vi "FTW-ActorTemplate-RT-TopLevel.vi"() -> ()   [LabVIEW 2013]
uses:
  source/actor/Instance/FTW-ActorInstance.lvclass
  source/actor/Message/Base/FTW-Message.lvclass
  source/actor/Instance/FTW-ActorInstance.lvclass/FTW-ActorInstance.ctl
  source/actor/JobSequencer/FTW-SEQ-Current.vi
  source/actor/Message/Request/FTW-Message-IncomingRequest.lvclass
  source/actor/Ether/FTW-Ether.lvclass
panel:
  in  "Process Stop Button":bool
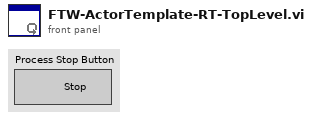
[diagram p1: front panel]
types:
  T1 = cluster{"Incoming Requests":refnum<event-registration>, "Local Messages":refnum<event-registration>, "Additional Registration Types":refnum<event-registration>}
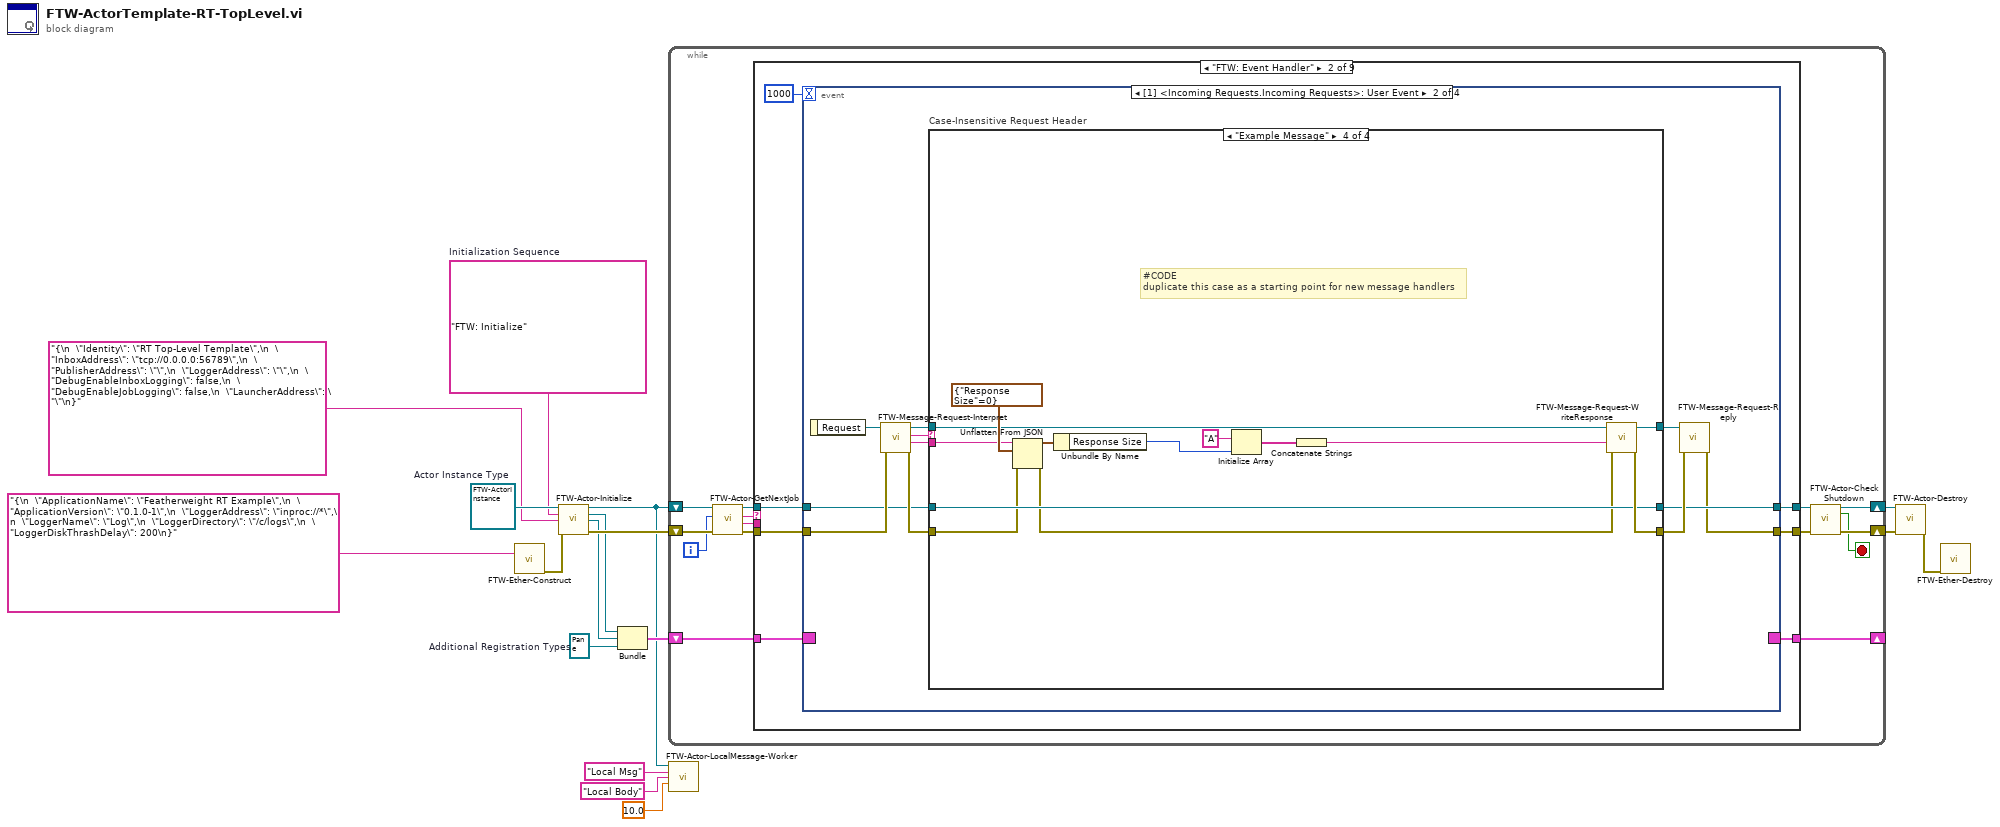
[diagram p0: block diagram]
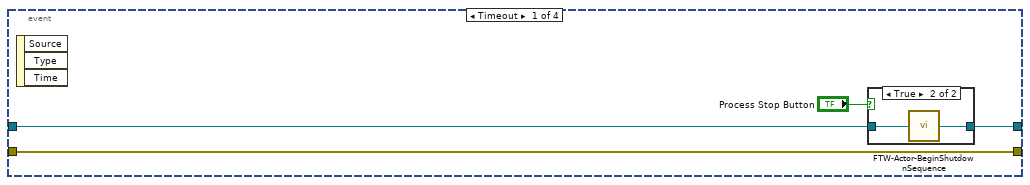
[diagram p3: hidden frame]
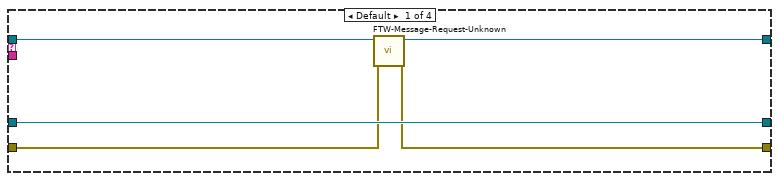
[diagram p5: hidden frame]
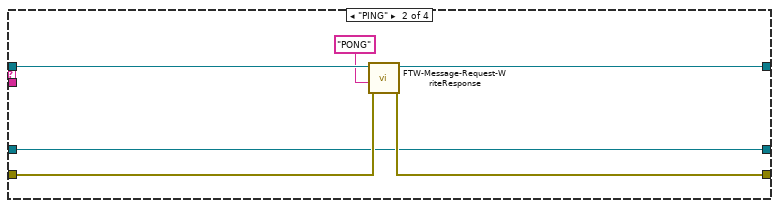
[diagram p6: hidden frame]
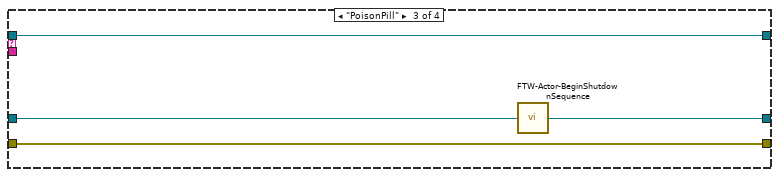
[diagram p7: hidden frame]
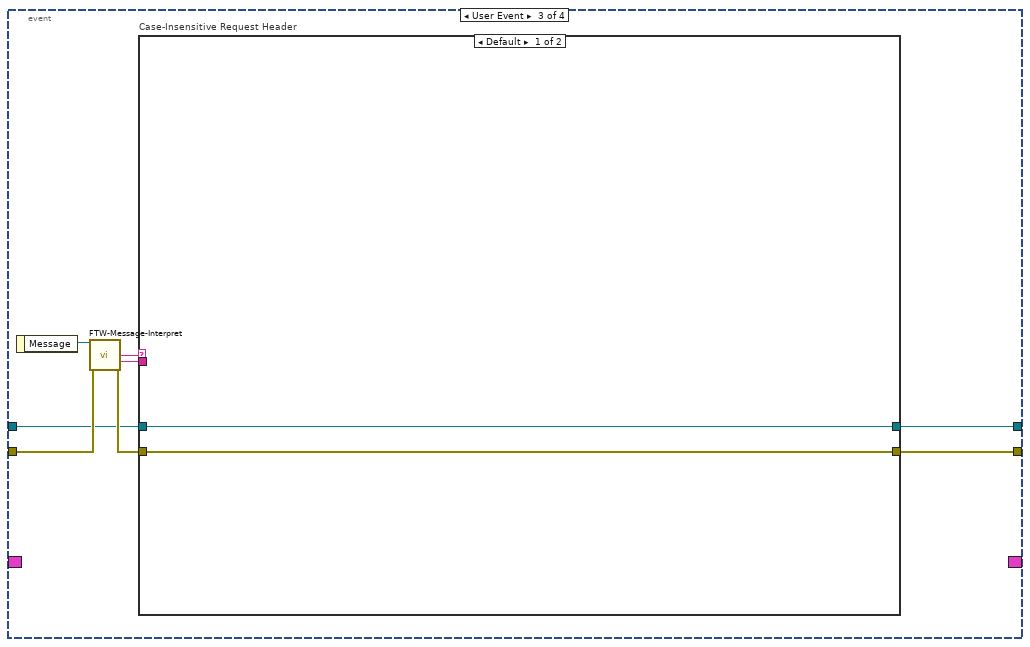
[diagram p8: hidden frame]
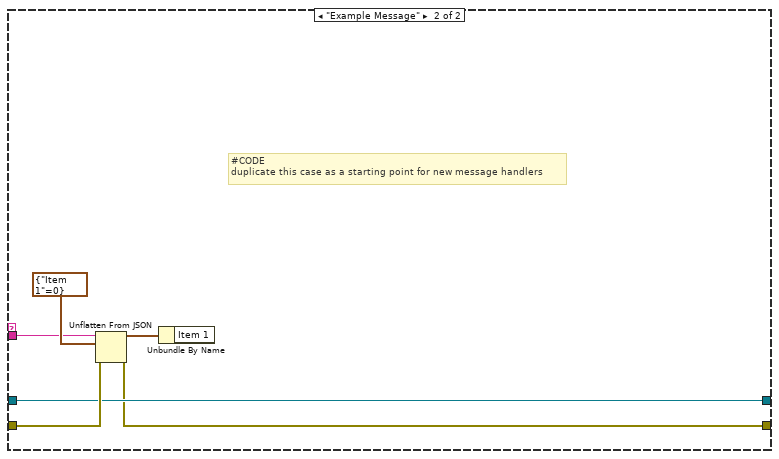
[diagram p9: hidden frame]
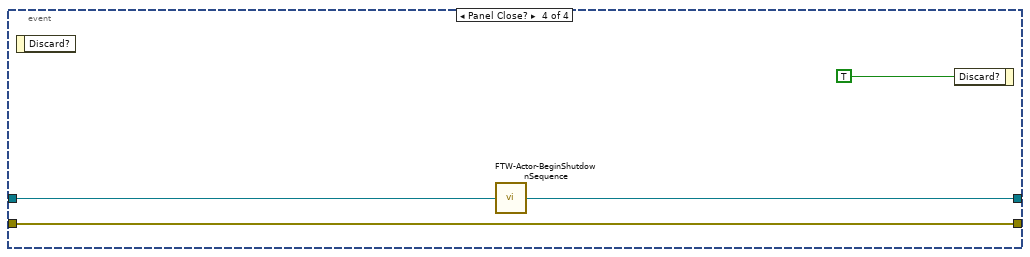
[diagram p10: hidden frame]
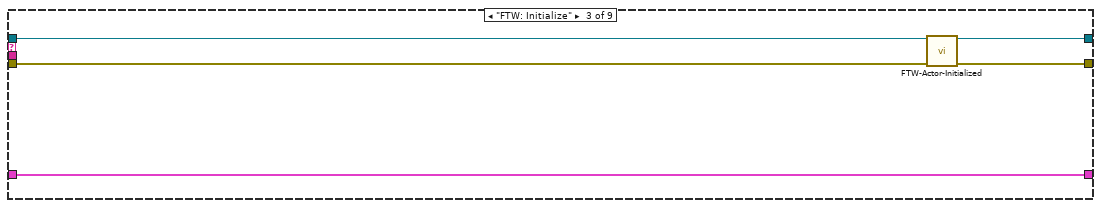
[diagram p11: hidden frame]
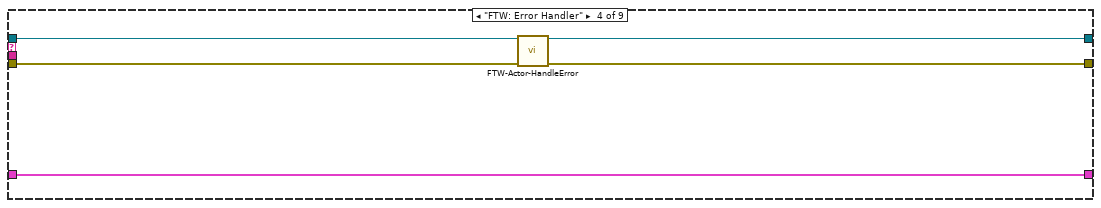
[diagram p12: hidden frame]
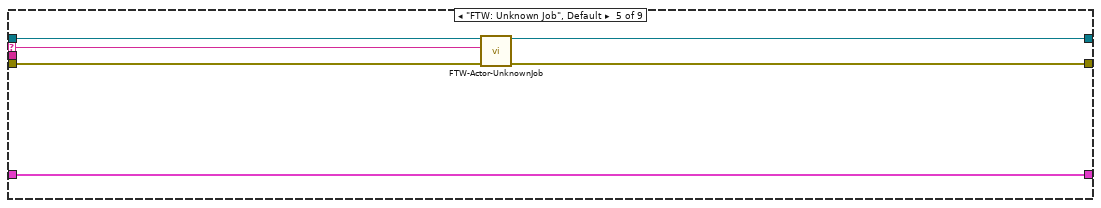
[diagram p13: hidden frame]
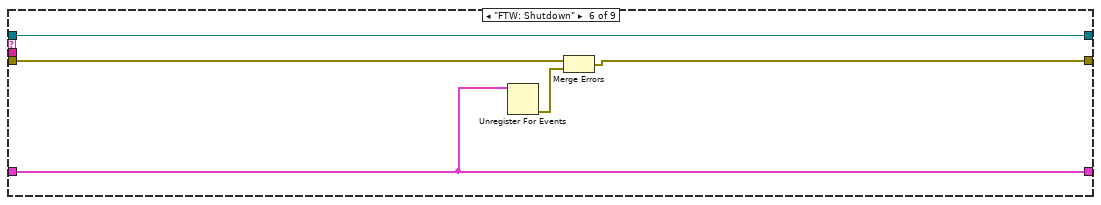
[diagram p14: hidden frame]
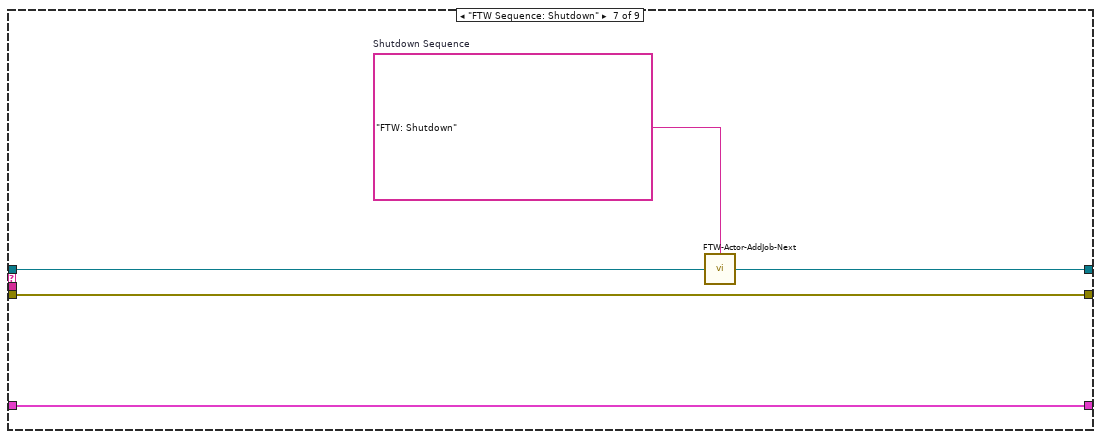
[diagram p15: hidden frame]
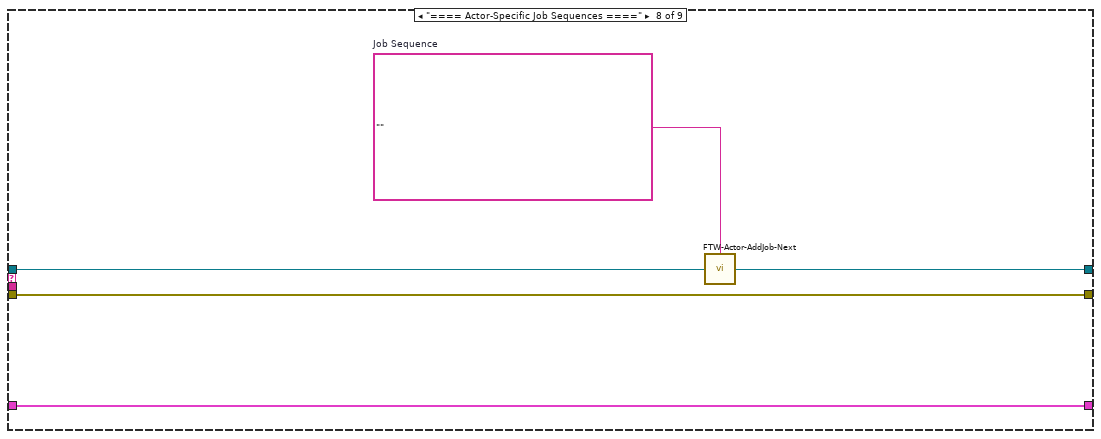
[diagram p16: hidden frame]
diagram:
  w8 = refnum<event-registration> refnum  # Additional Registration Types
  w13 = refnum<class "FTW-ActorInstance.lvclass"> refnum  # Actor Instance Type
  w12 = "FTW: Initialize"  # Initialization Sequence
  n1 = call "FTW-Ether-Construct.vi"("FTW Ether Configuration"="{\n  \"ApplicationName\": \"Featherweight RT Example\",\n  \"ApplicationVersion\": \"0.1.0-1\",\n  \"LoggerAddress\": \"inproc://*\",\n  \"LoggerName\": \"Log\",\n  \"LoggerDirectory\": \"/c/logs\",\n  \"LoggerDiskThrashDelay\": 200\n}") -> ("error out"=w7:errorcluster)  [unwired: 14 in]
  n2 = call-dynamic "FTW-Actor-Initialize.vi"("FTW Actor Instance Type"=w13, "Initialization Job Sequence"=w12, "Actor Instance Configuration"="{\n  \"Identity\": \"RT Top-Level Template\",\n  \"InboxAddress\": \"tcp://0.0.0.0:56789\",\n  \"PublisherAddress\": \"\",\n  \"LoggerAddress\": \"\",\n  \"DebugEnableInboxLogging\": false,\n  \"DebugEnableJobLogging\": false,\n  \"LauncherAddress\": \"\"\n}" ("FTW Actor Instance Configuration"), "error in"=w7) -> ("FTW Actor Instance"=w4:refnum<class "FTW-ActorInstance.lvclass">, "Incoming Requests"=w9:refnum<event-registration>, "Local Messages"=w5:refnum<event-registration>, "error out"=w14:errorcluster)  [unwired: 8 in]
  n3 = Bundle("Incoming Requests"=w9, "Local Messages"=w5, "Additional Registration Types"=w8) -> (w11:T1)  [unwired: 1 in]
  n4 = while {
    shift-right: [w21] -> w16
    shift-left: w14 -> [w28]
    shift-right: [w18] -> _
    shift-left: w11 -> [w31]
    shift-right: [w23] -> w17
    shift-left: w4 -> [w30]
    i -> [w19]
    stop <- w20 stop-if-true
    n5 = call "FTW-Actor-GetNextJob.vi"("error in"=w28, "Jobs Performed"=w19, "FTW Actor Instance"=w30) -> ("error out"=w27:errorcluster, "Job Data"=w25:string, "Job Name"=w26:string, "FTW Actor Instance out"=w29:refnum<class "FTW-ActorInstance.lvclass">)  [unwired: 5 in]
    n6 = case shown="\"FTW: Event Handler\"" w26 {
      selector: w26 -> [_ _ _ _ w118 _ _ _ _]
      tunnel: [w33 w41 w108 w113 w121 w127 w132 w137 w141] -> w22
      tunnel: w27 -> [w33 w40 w111 w115 w122 w128 w132 w137 w141]
      tunnel: w31 -> [w34 w36 w112 w117 w123 w124 w133 w138 w140]
      tunnel: [w34 w39 w112 w117 w123 w124 w133 w138 w140] -> w18
      tunnel: w25 -> [_ _ _ _ _ _ _ _ _]
      tunnel: [w32 w38 w109 w114 w119 w125 w130 w135 w139] -> w24
      tunnel: w29 -> [w32 w37 w110 w116 w120 w125 w131 w136 w139]
      frame "==== Featherweight Framework Jobs ====" {
      }
      frame "FTW: Event Handler" {
        n7 = event shown="[1] <Incoming Requests.Incoming Requests>: User Event" {
          selector: w36 -> [_ _ _ _]
          dyn-events: [_ _ _ _] -> w39
          timeout: 1000 -> [_ _ _ _]
          tunnel: [w45 w51 w92 w106] -> w41
          tunnel: w40 -> [w45 w57 w93 w106]
          tunnel: [w43 w55 w91 w104] -> w38
          tunnel: w37 -> [w44 w54 w90 w105]
          event Timeout {
            n8 = event-data() -> ()  [unwired: 1 in, 3 out]
            n9 = case shown="True" "Process Stop Button" {
              tunnel: w44 -> [w46 w48]
              tunnel: [w46 w47] -> w43
              frame False {
              }
              frame True {
                n10 = call "FTW-Actor-BeginShutdownSequence.vi"("FTW Actor Instance"=w48) -> ("FTW Actor Instance out"=w47:refnum<class "FTW-ActorInstance.lvclass">)  [unwired: 3 in]
              }
            }
          }
          event User Event {
            n11 = event-data() -> ("Request"=w58:refnum<class "FTW-Message-IncomingRequest.lvclass">)  [unwired: 1 in]
            n12 = call "FTW-Message-Request-Interpret.vi"("error in"=w57, "FTW Incoming Request"=w58) -> ("error out"=w59:errorcluster, "Request Body"=w49:string, "Request Header"=w53:string, "FTW Incoming Request out"=w52:refnum<class "FTW-Message-IncomingRequest.lvclass">)  [unwired: 6 in]
            n13 = case "Case-Insensitive Request Header" shown="\"Example Message\"" w53 {
              tunnel: [w62 w68 w73 w87] -> w56
              tunnel: w59 -> [w63 w69 w73 w75]
              tunnel: [w64 w67 w74 w85] -> w55
              tunnel: w54 -> [w64 w67 w72 w85]
              tunnel: w52 -> [w61 w70 w71 w77]
              tunnel: [w60 w66 w71 w86] -> w50
              tunnel: w49 -> [_ _ _ w76]
              frame Default {
                n14 = call "FTW-Message-Request-Unknown.vi"("error in"=w63, "FTW Incoming Request"=w61) -> ("error out"=w62:errorcluster, "FTW Incoming Request Out"=w60:refnum<class "FTW-Message-IncomingRequest.lvclass">)  [unwired: 8 in]
              }
              frame "PING" {
                n15 = call "FTW-Message-Request-WriteResponse.vi"("error in"=w69, "Response Body"="PONG" ("Response Header"), "FTW Incoming Request"=w70) -> ("error out"=w68:errorcluster, "FTW Incoming Request out"=w66:refnum<class "FTW-Message-IncomingRequest.lvclass">)  [unwired: 7 in]
              }
              frame "PoisonPill" {
                n16 = call "FTW-Actor-BeginShutdownSequence.vi"("FTW Actor Instance"=w72) -> ("FTW Actor Instance out"=w74:refnum<class "FTW-ActorInstance.lvclass">)  [unwired: 3 in]
              }
              frame "Example Message" {
                # "#CODE\nduplicate this case as a starting point for new message handlers"
                n17 = Unflatten From JSON(JSON string=w76, type and defaults=cluster{"Response Size":i32} {"Response Size"=0}, error in (no error)=w75) -> (value=w82:cluster{"Response Size":i32}, error out=w84:errorcluster)  [unwired: 4 in]
                n18 = Unbundle By Name(w82) -> ("Response Size"=w81:i32)
                n19 = Initialize Array("A", w81) -> (w79:string[])
                n20 = Concatenate Strings(w79) -> (w78:string)
                n21 = call "FTW-Message-Request-WriteResponse.vi"("error in"=w84, "Response Body"=w78, "FTW Incoming Request"=w77) -> ("error out"=w87:errorcluster, "FTW Incoming Request out"=w86:refnum<class "FTW-Message-IncomingRequest.lvclass">)  [unwired: 7 in]
              }
            }
            n22 = call "FTW-Message-Request-Reply.vi"("error in"=w56, "FTW Incoming Request"=w50) -> ("error out"=w51:errorcluster)  [unwired: 8 in, 1 out]
          }
          event User Event {
            n23 = event-data() -> ("Message"=w94:refnum<class "FTW-Message.lvclass">)  [unwired: 1 in]
            n24 = call-dynamic "FTW-Message-Interpret.vi"("FTW Message"=w94, "error in"=w93) -> ("Message Header"=w89:string, "Message Body"=w88:string, "error out"=w95:errorcluster)  [unwired: 9 in, 2 out]
            n25 = case "Case-Insensitive Request Header" shown="Default" w89 {
              tunnel: [w96 w101] -> w92
              tunnel: w95 -> [w96 w103]
              tunnel: [w97 w102] -> w91
              tunnel: w90 -> [w97 w102]
              tunnel: w88 -> [_ w98]
              frame Default {
              }
              frame "Example Message" {
                # "#CODE\nduplicate this case as a starting point for new message handlers"
                n26 = Unflatten From JSON(JSON string=w98, type and defaults=cluster{"Item 1":i32} {"Item 1"=0}, error in (no error)=w103) -> (value=w99:cluster{"Item 1":i32}, error out=w101:errorcluster)  [unwired: 4 in]
                n27 = Unbundle By Name(w99) -> ()  [unwired: 1 out]
              }
            }
          }
          event Panel Close? {
            n28 = event-data() -> ()  [unwired: 1 in, 1 out]
            n29 = call "FTW-Actor-BeginShutdownSequence.vi"("FTW Actor Instance"=w105) -> ("FTW Actor Instance out"=w104:refnum<class "FTW-ActorInstance.lvclass">)  [unwired: 3 in]
            n30 = event-data("Discard?"=TRUE) -> ()  [unwired: 1 in, 1 out]
          }
        }
      }
      frame "FTW: Initialize" {
        n31 = call-dynamic "FTW-Actor-Initialized.vi"("FTW Actor Instance"=w110, "error in"=w111) -> ("FTW Actor Instance out"=w109:refnum<class "FTW-ActorInstance.lvclass">, "error out"=w108:errorcluster)  [unwired: 12 in]
      }
      frame "FTW: Error Handler" {
        n32 = call-dynamic "FTW-Actor-HandleError.vi"("FTW Actor Instance"=w116, "error in"=w115) -> ("FTW Actor Instance out"=w114:refnum<class "FTW-ActorInstance.lvclass">, "error out"=w113:errorcluster)  [unwired: 11 in, 1 out]
      }
      frame "FTW: Unknown Job", Default {
        n33 = call-dynamic "FTW-Actor-UnknownJob.vi"("FTW Actor Instance"=w120, "Unknown Job"=w118, "error in"=w122) -> ("FTW Actor Instance out"=w119:refnum<class "FTW-ActorInstance.lvclass">, "error out"=w121:errorcluster)  [unwired: 11 in]
      }
      frame "FTW: Shutdown" {
        n34 = Unregister For Events(event registration refnum=w124) -> (error out=w126:errorcluster)  [unwired: 1 in]
        n35 = Merge Errors(w128, w126) -> (w127:errorcluster)
      }
      frame "FTW Sequence: Shutdown" {
        w129 = "FTW: Shutdown"  # Shutdown Sequence
        n36 = call "FTW-Actor-AddJob-Next.vi"("Add Next in Job Queue"=w129, "FTW Actor Instance"=w131) -> ("FTW Actor Instance out"=w130:refnum<class "FTW-ActorInstance.lvclass">)  [unwired: 2 in]
      }
      frame "==== Actor-Specific Job Sequences ====" {
        w134 = ""  # Job Sequence
        n37 = call "FTW-Actor-AddJob-Next.vi"("Add Next in Job Queue"=w134, "FTW Actor Instance"=w136) -> ("FTW Actor Instance out"=w135:refnum<class "FTW-ActorInstance.lvclass">)  [unwired: 2 in]
      }
      frame "==== Actor-Specific Jobs ====" {
      }
    }
    n38 = call "FTW-Actor-CheckShutdown.vi"("FTW Actor Instance"=w24, "error in"=w22) -> ("FTW Actor Instance out"=w23:refnum<class "FTW-ActorInstance.lvclass">, "Shutdown?"=w20:bool, "error out"=w21:errorcluster)  [unwired: 11 in]
  }
  n39 = call-dynamic "FTW-Actor-LocalMessage-Worker.vi"("FTW-ActorInstance In"=w4, "Message Header"="Local Msg", "Message Body"="Local Body", "Send Rate"=10.0) -> ()  [unwired: 11 in, 1 out]
  n40 = call-dynamic "FTW-Actor-Destroy.vi"("FTW Actor Instance"=w17, "error in"=w16) -> ("error out"=w15:errorcluster)  [unwired: 13 in]
  n41 = call "FTW-Ether-Destroy.vi"("error in"=w15) -> ()  [unwired: 14 in, 1 out]
